vi "Save LVClass.vi"(8 "error in (no error)":errorcluster, 10 "Path":path, 11 "LVClassLibrary in":refnum<vi>) -> (0 "error out":errorcluster, 3 "LVClassLibrary out":refnum<vi>)   [LabVIEW 2019, in "gRPC Scripting Tools.lvlib"]
uses:
  gRPC Scripting Tools.lvlib
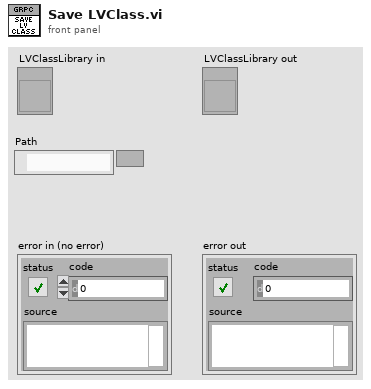
[diagram p1: front panel]
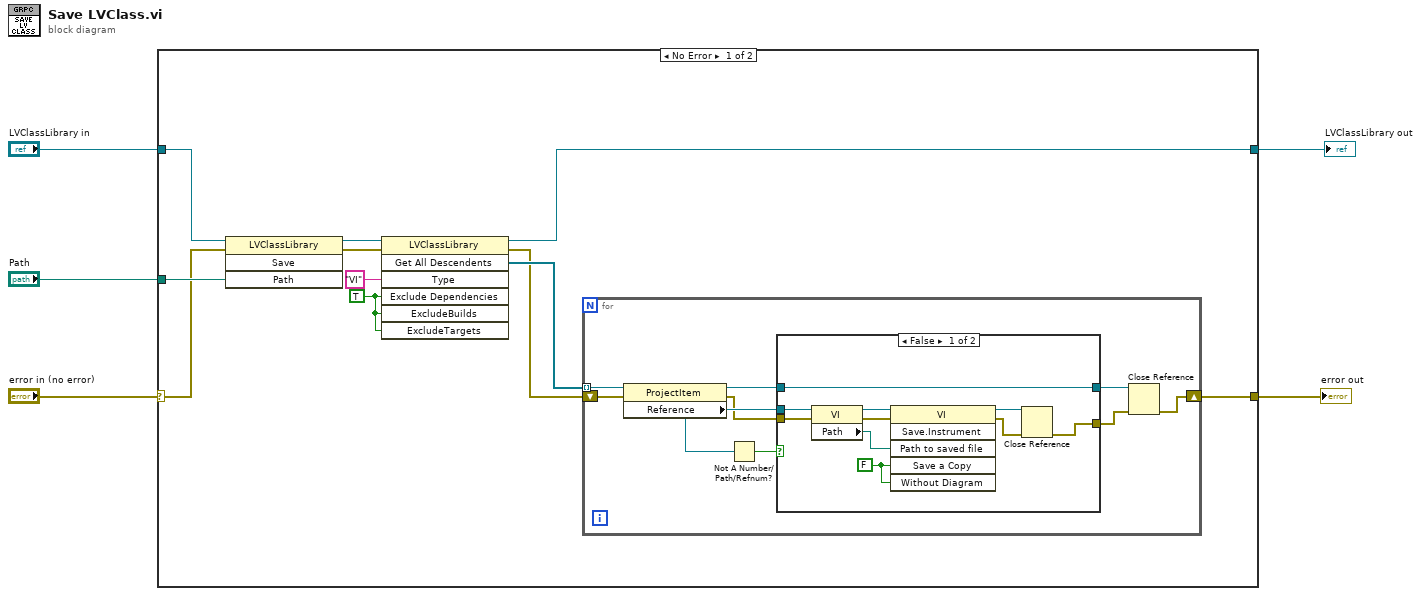
[diagram p0: block diagram]
diagram:
  n1 = case shown="No Error" "error in (no error)" {
    selector: "error in (no error)" -> [w8 w38]
    tunnel: "LVClassLibrary in" -> [w16 w39]
    tunnel: "Path" -> [w15 _]
    tunnel: [w10 w39] -> w3
    tunnel: [w9 w38] -> w2
    frame No Error {
      w6 = TRUE ("ExcludeDependencies")
      n2 = invoke class="LVClassLibrary" method="Save"(reference=w16, error in=w8, "Path"=w15) -> (reference out=w12:refnum<vi>, error out=w11:errorcluster)  [unwired: 1 in, 2 out]
      n3 = invoke class="LVClassLibrary" method="Get All Descendents"(reference=w12, error in=w11, "Type"="VI", "Exclude Dependencies"=w6, "ExcludeBuilds"=w6, "ExcludeTargets"=w6) -> (reference out=w10:refnum<vi>, error out=w13:errorcluster, "All Descendents"=w14:refnum<vi>[])  [unwired: 1 in, 4 out]
      n4 = for {
        tunnel: w14 -> [w25] mode=indexing
        shift-right: [w17] -> w9
        shift-left: w13 -> [w24]
        n5 = property class="ProjectItem"(reference=w25, error in=w24) -> (reference out=w23:refnum<vi>, error out=w20:errorcluster, "Reference"=w21:refnum<vi>)
        n6 = Not A Number/Path/Refnum?(number/path/refnum=w21) -> (NaN/Path/Refnum?=w22:bool)
        n7 = case shown="False" w22 {
          tunnel: [w29 w36] -> w18
          tunnel: w23 -> [w28 w37]
          tunnel: w21 -> [w30 _]
          tunnel: [w28 w37] -> w19
          tunnel: w20 -> [w27 w36]
          frame False {
            w33 = FALSE ("Save a Copy")
            n8 = property class="VI"(reference=w30, error in=w27) -> (reference out=w35:refnum<vi>, error out=w34:errorcluster, "Path"=w26:path)
            n9 = invoke class="VI" method="Save.Instrument"(reference=w35, error in=w34, "Path to saved file"=w26, "Save a Copy"=w33, "Without Diagram"=w33) -> (reference out=w32:refnum<vi>, error out=w31:errorcluster)  [unwired: 1 in, 4 out]
            n10 = Close Reference(reference=w32, error in (no error)=w31) -> (error out=w29:errorcluster)
          }
          frame True {
          }
        }
        n11 = Close Reference(reference=w19, error in (no error)=w18) -> (error out=w17:errorcluster)
      }
    }
    frame Error {
    }
  }
  "LVClassLibrary out" <- w3
  "error out" <- w2
